vi "pickup.vi"(0 "Picking up Angle":dbl(knob) scale=-1.0..1.0, 1 "isFull?":bool, 3 "frisbee?":bool, 5 "Arm ref num":string="My Motor RefNum", 7 "Speed":dbl, 9 "Up":bool, 11 "Down":bool, 12 "Mode":bool) -> ()   [LabVIEW 2012]
panel:
  out "Enum":enum16{"Up", "Down", "Stop"}(ring)
  out "IsUp?":bool
  out "IsDown?":bool
  in  "stop":bool
  out "Manual Mode":bool
  out "Auto Mode":bool
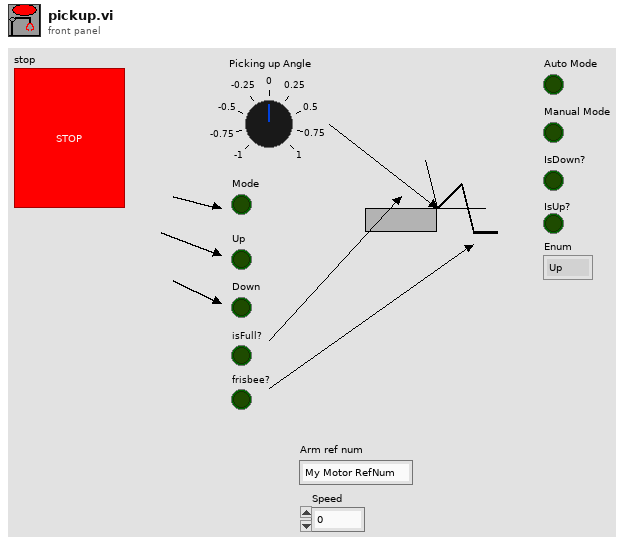
[diagram p1: front panel]
types:
  T1 = typedef "WPI_MotorControlDeviceRef.ctl" = cluster{"DeviceStatus":errorcluster, "Type":enum16{"PWM", "CAN"}, "PWM":cluster{"Digital Module":T2, "PWM Channel":T3, "DeadBand":T4}, "CAN":cluster{"Device Number":u8, "Control Mode":T5, "Semaphore":T6, "Max Vout":dbl}, "Invert":bool, "TransformRef":T7, "InvTransformRef":T7}
  T2 = typedef "FPGA_TypedefDigitalModule.ctl" = enum16{"Digital Module 1", "Digital Module 2"}
  T3 = typedef "FPGA_DIOPWMChannel.ctl" = enum8{"PWM 1", "PWM 2", "PWM 3", "PWM 4", "PWM 5", "PWM 6", "PWM 7", "PWM 8", "PWM 9", "PWM 10", "Invalid"}
  T4 = typedef "WPI_PWMDeadband.ctl" = cluster{"Name":string, "maxPositivePwm":i32, "minPositivePwm":i32, "centerPwm":i32, "maxNegativePwm":i32, "minNegativePwm":i32, "angularRange":u16}
  T5 = typedef "WPI_CANJaguar_ControlMode.ctl" = enum8{"Percent VBus", "Current", "Speed", "Position", "Voltage"}
  T6 = typedef "Semaphore RefNum" = refnum<k1>
  T7 = typedef "WPI_PWMTransform_ConPane.ctl" = refnum<vi>
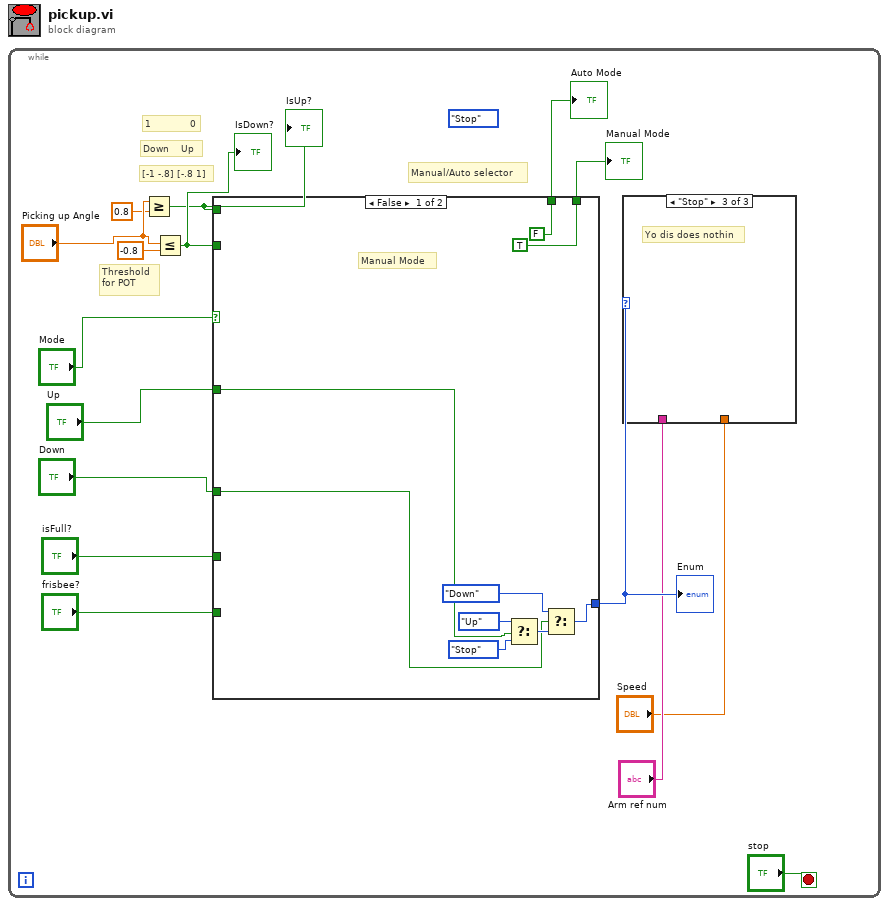
[diagram p0: block diagram]
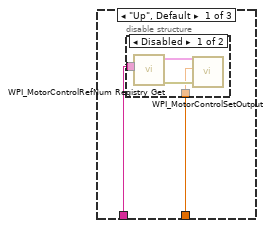
[diagram p2: hidden frame]
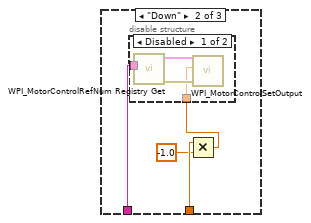
[diagram p4: hidden frame]
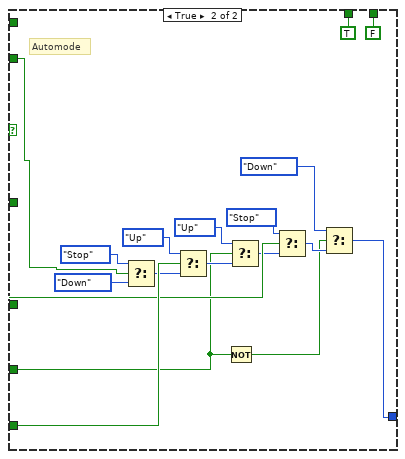
[diagram p6: hidden frame]
diagram:
  n1 = while {
    stop <- "stop" stop-if-true
    (unwired) enum16{"Up", "Down", "Stop"}."Stop"
    # "Manual/Auto selector"
    # "1             0"
    # "Threshold \nfor POT"
    # "Down    Up"
    # "[-1 -.8] [-.8 1]"
    n2 = Greater Or Equal?(x="Picking up Angle", y=0.8) -> (x >= y?=w2:bool)
    "IsUp?" <- w2
    n3 = Less Or Equal?(x="Picking up Angle", y=-0.8) -> (x <= y?=w4:bool)
    "IsDown?" <- w4
    n4 = case shown="False" "Mode" {
      tunnel: [TRUE ("Manual Mode") FALSE ("Manual Mode")] -> w14
      tunnel: [FALSE ("Manual Mode") TRUE ("Manual Mode")] -> w13
      tunnel: "Up" -> [w37 _]
      tunnel: "Down" -> [w31 _]
      tunnel: [w33 w43] -> w10
      tunnel: w4 -> [_ w55]
      tunnel: "frisbee?" -> [_ w52]
      tunnel: w2 -> [_ w48]
      tunnel: "isFull?" -> [_ w41]
      frame False {
        # "Manual Mode"
        n5 = Select(t=enum16{"Up", "Down", "Stop"}."Up", s=w37, f=enum16{"Up", "Down", "Stop"}."Stop") -> (s? t:f=w35:enum16{"Up", "Down", "Stop"})
        n6 = Select(t=enum16{"Up", "Down", "Stop"}."Down", s=w31, f=w35) -> (s? t:f=w33:enum16{"Up", "Down", "Stop"})
      }
      frame True {
        # "Automode"
        n7 = Select(t=enum16{"Up", "Down", "Stop"}."Stop", s=w55, f=enum16{"Up", "Down", "Stop"}."Down") -> (s? t:f=w51:enum16{"Up", "Down", "Stop"})
        n8 = Select(t=enum16{"Up", "Down", "Stop"}."Up", s=w52, f=w51) -> (s? t:f=w45:enum16{"Up", "Down", "Stop"})
        n9 = Not(x=w41) -> (.not. x?=w40:bool)
        n10 = Select(t=enum16{"Up", "Down", "Stop"}."Up", s=w41, f=w45) -> (s? t:f=w46:enum16{"Up", "Down", "Stop"})
        n11 = Select(t=enum16{"Up", "Down", "Stop"}."Stop", s=w48, f=w46) -> (s? t:f=w44:enum16{"Up", "Down", "Stop"})
        n12 = Select(t=enum16{"Up", "Down", "Stop"}."Down", s=w40, f=w44) -> (s? t:f=w43:enum16{"Up", "Down", "Stop"})
      }
    }
    "Auto Mode" <- w13
    "Manual Mode" <- w14
    "Enum" <- w10
    n13 = case shown="\"Stop\"" w10 {
      tunnel: "Arm ref num" -> [w18 w26 _]
      tunnel: "Speed" -> [w17 w25 _]
      frame "Up", Default {
        n14 = disable-structure shown="Disabled" {
          disable-tunnel: w18 -> [w20 _]
          disable-tunnel: w17 -> [w19 _]
          frame Disabled {
            n15 = call <vilib>:"WPI_MotorControlRefNum Registry Get.vi"("refnum name"=w20) -> ("error out"=w22:errorcluster, "MotorControlDevRef"=w21:T1)  [unwired: 9 in]
            n16 = call <vilib>:"WPI_MotorControlSetOutput.vi"("error in (no error)"=w22, "Output"=w19, "MotorControlDevRef"=w21) -> ()  [unwired: 6 in, 3 out]
          }
          frame Enabled {
          }
        }
      }
      frame "Down" {
        n17 = Multiply(x=w25, y=-1.0) -> (x*y=w24:dbl)
        n18 = disable-structure shown="Disabled" {
          disable-tunnel: w26 -> [w30 _]
          disable-tunnel: w24 -> [w27 _]
          frame Disabled {
            n19 = call <vilib>:"WPI_MotorControlRefNum Registry Get.vi"("refnum name"=w30) -> ("error out"=w29:errorcluster, "MotorControlDevRef"=w28:T1)  [unwired: 9 in]
            n20 = call <vilib>:"WPI_MotorControlSetOutput.vi"("error in (no error)"=w29, "Output"=w27, "MotorControlDevRef"=w28) -> ()  [unwired: 6 in, 3 out]
          }
          frame Enabled {
          }
        }
      }
      frame "Stop" {
        # "Yo dis does nothin"
      }
    }
  }
